vi "7-New OCU.vi"() -> ()   [LabVIEW 2010]
uses:
  4-High Neurons/4.0-Timing Badass.ctl
  7-OCU/7.0 GUI/7.0 Manual Mode Display.ctl
  6-OCU Neurons/6.1-UDP Saitek.ctl
  <vilib>/robotics/Controls/Compass Indicator/Compass Indicator.xctl
  7-OCU/7.0-OCU State.ctl
  7-OCU/7.0 GUI/7.0 Auto Mode Display.ctl
  7-OCU/7.0-Global.vi
panel:
  in  "Tab Control":T1(tab)
  out "7.0 Manual Mode GUI":T2 {"Speed (m/s)" scale=0.0..2.5; "Battery" scale=0.0..24.0; "6.1-Saitek Controller"."Right" scale=-32767.0..32767.0; "6.1-Saitek Controller"."Left" scale=-32767.0..32767.0; "6.1-Saitek Controller"."Yaw" scale=-32767.0..32767.0; "6.1-Saitek Controller"."Roll" scale=-32767.0..32767.0; "6.1-Saitek Controller"."Pitch" scale=-32767.0..32767.0}
  out "7.0 Auto Mode Display":T4 {"Speed (m/s)" scale=0.0..2.5; "Battery" scale=20.0..24.0}
  out "7.0 OCU State":T5
  out "GUI Heart Beat":T6
  in  "Shutdown":bool
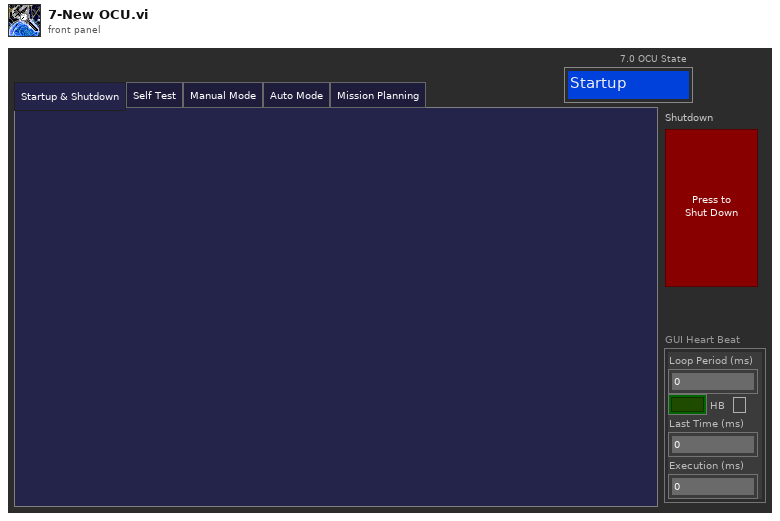
[diagram p1: front panel]
types:
  T1 = enum32{"Startup & Shutdown", "Self Test", "Manual Mode", "Auto Mode", "Mission Planning"}
  T2 = typedef "7.0 Manual Mode Display.ctl" = cluster{"6.1-Saitek Controller":T3, "Manual Override":bool, "Shutdown":bool, "Reset":bool, "Begin":bool, "Time":dbl, "Battery":dbl, "Speed (m/s)":dbl, "Heading":dbl}
  T3 = typedef "6.1-UDP Saitek.ctl" = cluster{"Trig":bool, "2":bool, "3":bool, "4":bool, "5":bool, "6":bool, "7":bool, "8":bool, "9":bool, "10":bool, "11":bool, "Pitch":i32, "Ang":bool[], "Wheel":dbl, "Roll":i32, "Yaw":i32, "Left":i32, "Right":i32}
  T4 = typedef "7.0 Auto Mode Display.ctl" = cluster{"Shutdown CMD":bool, "Time":dbl, "Battery":dbl, "Speed (m/s)":dbl, "Heading":dbl, "XY Graph":cluster{dbl, dbl}[], "Latitude":dbl, "Longitude":dbl, "Lattitude of Waypoint":dbl, "Longitude of Waypoint":dbl, "Distance to Waypoint":dbl, "Has Mission Def":bool}
  T5 = typedef "7.0-OCU State.ctl" = enum16{"Startup", "Self Test", "Manual Mode", "Auto Mode", "Plan Mission", "Shutdown"}
  T6 = typedef "4.0-Timing Badass.ctl" = cluster{"Loop Period (ms)":u32, "HB":bool, "Last Time (ms)":u32, "Execution (ms)":u32}
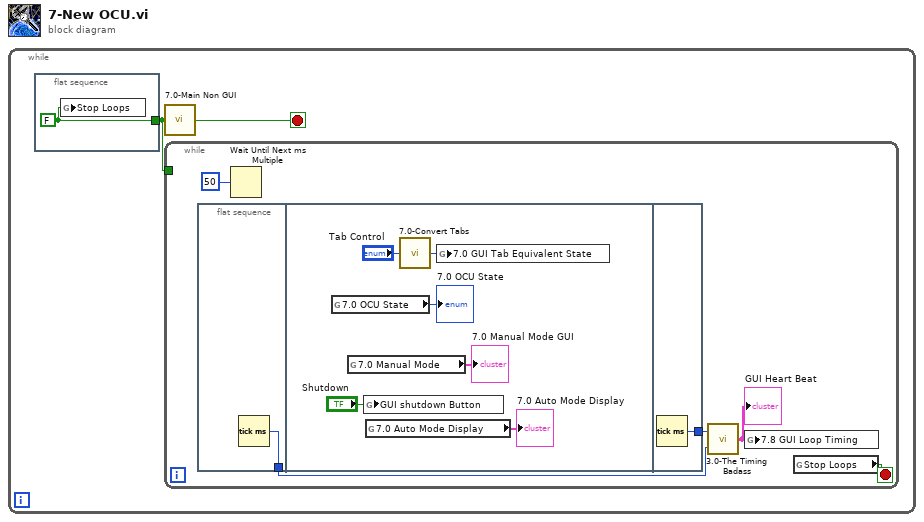
[diagram p0: block diagram]
diagram:
  n1 = while {
    stop <- w1 stop-if-true
    n2 = flat-sequence {
      tunnel: [w3] -> w2
      frame #0 {
        w3 = FALSE ("Stop Loops")
        n3 = global write "7.0-Global.vi" "Stop Loops"(w3) -> ()
      }
    }
    n4 = call "7.0-Main Non GUI.vi"("Begin (for Flow)"=w2) -> ("End Program"=w1:bool)
    n5 = while "7.0 GUI Loop" {
      tunnel: w2 -> [_]
      stop <- w7 stop-if-true
      n6 = flat-sequence {
        tunnel: [w9] -> w5
        tunnel: [w16] -> w6
        frame #0 {
          n7 = Tick Count (ms)() -> (millisecond timer value=w9:u32)
        }
        frame #1 {
          n8 = global read "7.0-Global.vi" "7.0 OCU State"() -> (→"7.0 OCU State":T5)
          n9 = global read "7.0-Global.vi" "7.0 Manual Mode"() -> (→"7.0 Manual Mode GUI":T2)
          n10 = global write "7.0-Global.vi" "GUI shutdown Button"("Shutdown") -> ()
          n11 = global read "7.0-Global.vi" "7.0 Auto Mode Display"() -> (→"7.0 Auto Mode Display":T4)
          n12 = call "7.0-Convert Tabs.vi"("Tab Control"="Tab Control") -> ("7.0 GUI Tab Equivalent State"=w10:T5)
          n13 = global write "7.0-Global.vi" "7.0 GUI Tab Equivalent State"(w10) -> ()
        }
        frame #2 {
          n14 = Tick Count (ms)() -> (millisecond timer value=w16:u32)
        }
      }
      n15 = Wait Until Next ms Multiple(millisecond multiple=u32 50) -> ()  [unwired: 1 out]
      n16 = call "3.0-The Timing Badass.vi"("Start"=w5, "End"=w6) -> ("Super Heart Beat"=w4:T6)
      "GUI Heart Beat" <- w4
      n17 = global write "7.0-Global.vi" "7.8 GUI Loop Timing"(w4) -> ()
      n18 = global read "7.0-Global.vi" "Stop Loops"() -> (w7:bool)
    }
  }
